vi "wykonajRuch.vi"(8 "error in (no error)":errorcluster, 9 "Lista komór":T1[](array[typedef]), 10 "Akcja":T2=enum."Sprawdź", 11 "LINX Resource in":T3) -> (0 "error out":errorcluster, 3 "LINX Resource out":T3)   [LabVIEW 2014]
uses:
  <vilib>/MakerHub/LINX/Private/Type Defs/LINX Ref.ctl
  <vilib>/MakerHub/LINX/Private/Type Defs/Platform.ctl
  <vilib>/MakerHub/LINX/Private/Type Defs/Interface.ctl
  <vilib>/MakerHub/LINX/Private/Device/Type Defs/LINX Device Config.ctl
  <vilib>/MakerHub/LINX/Private/Device/Type Defs/TCP Config.ctl
  <vilib>/MakerHub/LINX/Private/Device/Type Defs/Channels.ctl
  AkcjaRuchu.ctl
  wykonajRuchVIs/parametryKomorVIs/WyborKomory.ctl
  AkcjaGFV.ctl
  <vilib>/MakerHub/LINX/LMH-LINX.lvlib
  <vilib>/MakerHub/LINX/Private/Device/Device.lvlib
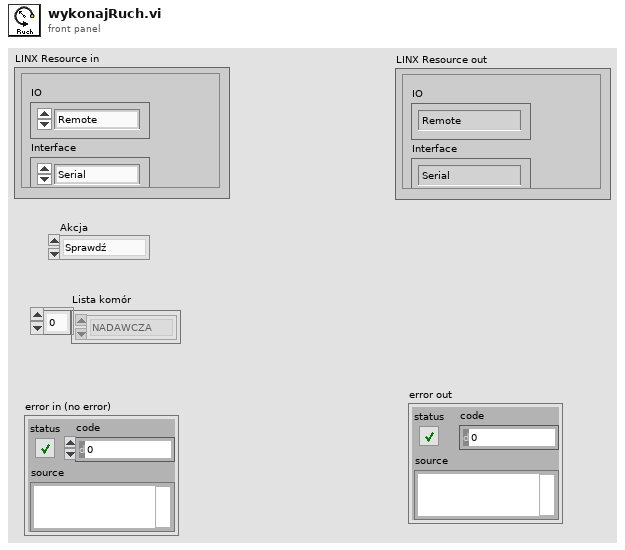
[diagram p1: front panel]
types:
  T1 = typedef "WyborKomory.ctl" = enum16{"NADAWCZA", "ODBIORCZA"}
  T2 = typedef "AkcjaRuchu.ctl" = enum16{"Init", "Reset ramienia", "Przygotuj listę", "Sprawdź", "Koniec"}
  T3 = typedef "LMH-LINX.lvlib/LINX Ref.ctl" = cluster{"IO":T4, "Interface":T5, "LINX Device Config":T6}
  T4 = typedef "LMH-LINX.lvlib/Platform.ctl" = enum16{"Remote", "Local"}
  T5 = typedef "LMH-LINX.lvlib/Interface.ctl" = enum16{"Serial", "TCP"}
  T6 = typedef "LMH-LINX.lvlib/Device.lvlib/LINX Device Config.ctl" = cluster{"Interface":T5, "COM Port":refnum<visa-resource-name>, "TCP Configuration":T7, "Device Family":u8, "Device ID":u8, "Device Name":string, "TCP Ref":refnum<k5>, "Channels":T8}
  T7 = typedef "LMH-LINX.lvlib/Device.lvlib/TCP Config.ctl" = cluster{"IP Address":string, "Port":u16}
  T8 = typedef "LMH-LINX.lvlib/Channels.ctl" = cluster{"DI":u8[], "DO":u8[], "AI":u8[], "AO":u8[], "PWM":u8[], "QE":u8[], "UART":u8[], "I2C 2":u8[], "SPI":u8[], "CAN":u8[], "Servo":u8[], "AI Ref (V)":dbl, "AI Resolution (Bits)":u8, "AO Ref (V)":dbl, "AO Resolution (Bits)":u8}
  T9 = typedef "AkcjaGFV.ctl" = enum16{"Czytaj", "Zapisz", "Reset"}
  T10 = typedef "WyjsciaParametry.ctl" = cluster{"Nad. lewo":bool, "Nad.  prawo":bool, "Nad.  gora":bool, "Nad. doł":bool, "Dzialanie":bool, "Pomiar":bool, "Odb. lewo":bool, "Odb.  prawo":bool, "Odb.  gora":bool, "Odb. dol":bool, "Pozostalo punktow":i32, "Nad. elewacja":i32, "Nad. azymut":i32, "Odb. elewacja":i32, "Odb. azymut":i32, "TCP Error":bool, "TCP Error Code":i32, "LINX Error":bool, "LINX Error Code":i32, "Nastepny elewacja":i32, "Nastepny azymut":i32, "Coords Error":bool, "Inicjalizacja pozycji":bool}
  T11 = typedef "RuchPoziomy.ctl" = enum16{"PRACA RĘCZNA", "LEWO", "PRAWO", "WYŁ."}
  T12 = typedef "RuchPionowy.ctl" = enum16{"WYŁ.", "GÓRA", "Dӣ", "PRACA RĘCZNA"}
  T13 = typedef "WejsciaParametry.ctl" = cluster{"LEWO":bool, "PRAWO":bool, "GORA":bool, "DOL":bool, "Praca reczna":bool, "Stop":bool, "Start":bool, "Komora":bool, "Wyjscie":bool, "Rodzaj pomiarow":T14, "Czas pomiaru [s]":dbl, "Czas inicjalizacji ramion [s]":dbl, "Liczba punktów":i32, "Liczba płaszczyzn":i32}
  T14 = typedef "RodzajPomiarow.ctl" = enum16{"Izolacyjność Akustyczna ISO 10140", "Losowanie punktów", "Sekwencja testowa"}
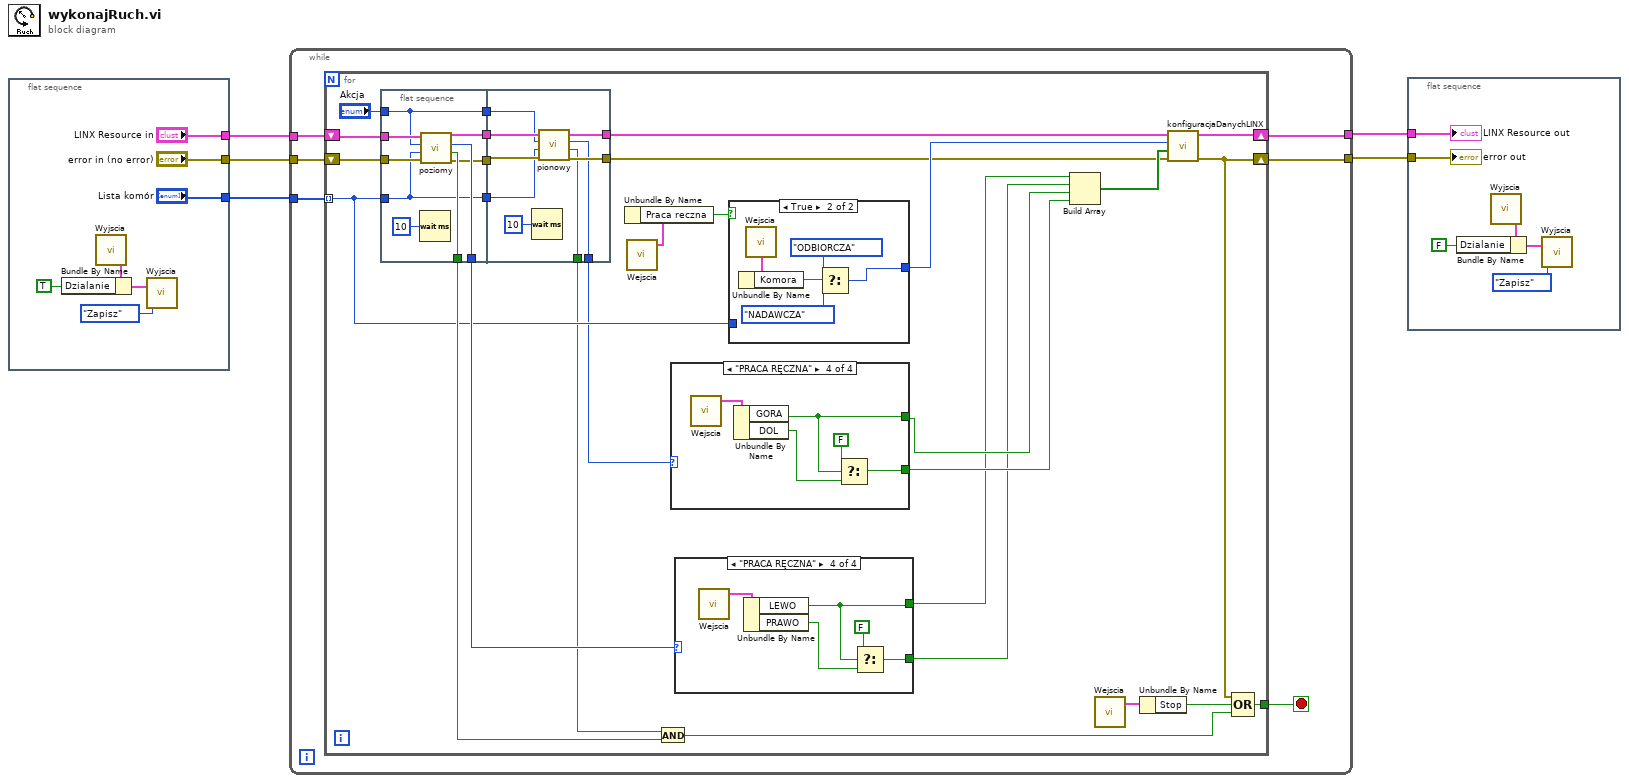
[diagram p0: block diagram]
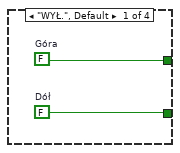
[diagram p3: hidden frame]
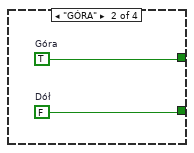
[diagram p4: hidden frame]
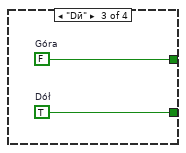
[diagram p5: hidden frame]
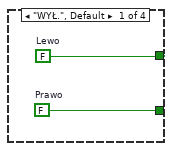
[diagram p6: hidden frame]
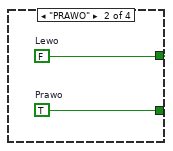
[diagram p7: hidden frame]
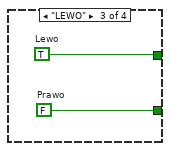
[diagram p8: hidden frame]
diagram:
  n1 = flat-sequence {
    tunnel: ["error in (no error)"] -> w1
    tunnel: ["LINX Resource in"] -> w5
    tunnel: ["Lista komór"] -> w2
    frame #0 {
      n2 = call "Wyjscia.vi"() -> ("Wyjście"=w9:T10)  [unwired: 5 in]
      n3 = Bundle By Name(cluster=w9, "Dzialanie"=TRUE ("Wejście")) -> (w7:T10)
      n4 = call "Wyjscia.vi"("Akcja"=AkcjaGFV."Zapisz", "Wejście"=w7) -> ()  [unwired: 3 in, 1 out]
    }
  }
  n5 = while {
    tunnel: w5 -> [w17]
    tunnel: w1 -> [w18]
    tunnel: [w15] -> w3
    tunnel: [w14] -> w4
    tunnel: w2 -> [w13]
    stop <- w16 stop-if-true
    n6 = for {
      tunnel: [w35] -> w16
      tunnel: w13 -> [w29] mode=indexing
      shift-right: [w33] -> w14
      shift-left: w18 -> [w45]
      shift-right: [w34] -> w15
      shift-left: w17 -> [w43]
      n7 = flat-sequence {
        tunnel: w45 -> [w55]
        tunnel: w43 -> [w53]
        tunnel: "Akcja" -> [w48]
        tunnel: [w52] -> w42
        tunnel: [w51] -> w41
        tunnel: w29 -> [w49]
        tunnel: [w54] -> w27
        tunnel: [w50] -> w26
        tunnel: [w49] -> w20
        tunnel: [w48] -> w19
        tunnel: w27 -> [w64]
        tunnel: w26 -> [w63]
        tunnel: [w62] -> w25
        tunnel: [w61] -> w24
        tunnel: [w60] -> w22
        tunnel: [w59] -> w21
        tunnel: w20 -> [w58]
        tunnel: w19 -> [w57]
        frame #0 {
          n8 = Wait (ms)(milliseconds to wait=u32 10 ("dt pętli")) -> ()  [unwired: 1 out]
          n9 = call "poziomy.vi"("error in (no error)"=w55, "Wybór komory"=w49, "Akcja"=w48, "LINX Resource in"=w53) -> ("error out"=w50:errorcluster, "KONIEC"=w51:bool, "Aktualny stan"=w52:T11, "LINX Resource out"=w54:T3)  [unwired: 2 in]
        }
        frame #1 {
          n10 = Wait (ms)(milliseconds to wait=u32 10 ("dt pętli")) -> ()  [unwired: 1 out]
          n11 = call "pionowy.vi"("error in"=w63, "Wybór komory"=w58, "Akcja"=w57, "LINX Resource in"=w64) -> ("error out"=w61:errorcluster, "KONIEC"=w60:bool, "Aktualny stan"=w59:T12, "LINX Resource out"=w62:T3)  [unwired: 2 in]
        }
      }
      n12 = call "Wejscia.vi"() -> ("Wyjście"=w31:T13)  [unwired: 5 in]
      n13 = Unbundle By Name(w31) -> ("Praca reczna"=w30:bool)
      n14 = And(x=w22, y=w41) -> (x .and. y?=w36:bool)
      n15 = case shown="\"PRACA RĘCZNA\"" w21 {
        tunnel: [w72 w74 w76 w78] -> w40
        tunnel: [w71 w73 w75 w81] -> w44
        frame "WYŁ.", Default {
          w71 = FALSE  # Dół
          w72 = FALSE  # Góra
        }
        frame "GÓRA" {
          w73 = FALSE  # Dół
          w74 = TRUE  # Góra
        }
        frame "Dӣ" {
          w75 = TRUE  # Dół
          w76 = FALSE  # Góra
        }
        frame "PRACA RĘCZNA" {
          n16 = call "Wejscia.vi"() -> ("Wyjście"=w79:T13)  [unwired: 5 in]
          n17 = Unbundle By Name(w79) -> ("GORA"=w78:bool, "DOL"=w77:bool)
          n18 = Select(t=FALSE, s=w78, f=w77) -> (s? t:f=w81:bool)
        }
      }
      n19 = case shown="\"PRACA RĘCZNA\"" w42 {
        tunnel: [w83 w85 w87 w89] -> w39
        tunnel: [w82 w84 w86 w92] -> w38
        frame "WYŁ.", Default {
          w82 = FALSE  # Prawo
          w83 = FALSE  # Lewo
        }
        frame "PRAWO" {
          w84 = TRUE  # Prawo
          w85 = FALSE  # Lewo
        }
        frame "LEWO" {
          w86 = FALSE  # Prawo
          w87 = TRUE  # Lewo
        }
        frame "PRACA RĘCZNA" {
          n20 = call "Wejscia.vi"() -> ("Wyjście"=w90:T13)  [unwired: 5 in]
          n21 = Unbundle By Name(w90) -> ("LEWO"=w89:bool, "PRAWO"=w88:bool)
          n22 = Select(t=FALSE, s=w89, f=w88) -> (s? t:f=w92:bool)
        }
      }
      n23 = case shown="True" w30 {
        tunnel: [w65 w70] -> w28
        tunnel: w29 -> [w65 _]
        frame False {
        }
        frame True {
          n24 = call "Wejscia.vi"() -> ("Wyjście"=w69:T13)  [unwired: 5 in]
          n25 = Unbundle By Name(w69) -> ("Komora"=w68:bool)
          n26 = Select(t=WyborKomory."ODBIORCZA" ("Wybór komory"), s=w68, f=WyborKomory."NADAWCZA" ("Wybór komory")) -> (s? t:f=w70:T1)
        }
      }
      n27 = Build Array(w39, w38, w40, w44) -> (w32:bool[])
      n28 = call "Wejscia.vi"() -> ("Wyjście"=w46:T13)  [unwired: 5 in]
      n29 = Unbundle By Name(w46) -> ("Stop"=w37:bool)
      n30 = call "konfiguracjaDanychLINX.vi"("Error In"=w24, "Kierunki"=w32, "Wybór komory"=w28, "LINX Resource"=w25) -> ("Error Out"=w33:errorcluster, "LINX Out"=w34:T3)  [unwired: 6 in]
      n31 = Compound Arithmetic op=OR(w33, w37, w36) -> (w35:bool)
    }
  }
  n32 = flat-sequence {
    tunnel: w4 -> [w93]
    tunnel: w3 -> [w98]
    frame #0 {
      n33 = call "Wyjscia.vi"() -> ("Wyjście"=w96:T10)  [unwired: 5 in]
      n34 = Bundle By Name(cluster=w96, "Dzialanie"=FALSE ("Wejście")) -> (w94:T10)
      n35 = call "Wyjscia.vi"("Akcja"=AkcjaGFV."Zapisz", "Wejście"=w94) -> ()  [unwired: 3 in, 1 out]
      "error out" <- w93
      "LINX Resource out" <- w98
    }
  }
